vi "SubPanel - Power Analysis.vi"() -> ()   [LabVIEW 2021]
uses:
  <vilib>/Analysis/5stat.llb/RMS (DBL).vi
  <vilib>/Analysis/NI_AALPro.lvlib
panel:
  out "error out":errorcluster
  in  "error in":errorcluster
  in  "Samples per Channel":i32
  out "I Phase L3":dbl format="%#.3g"
  out "I Phase L2":dbl format="%#.3g"
  out "I Phase L1":dbl format="%#.3g"
  out "Instantaneus Currents":dbl[][](graph)
  out "P/S Total":dbl format="%#.3g"
  out "Q Total":dbl format="%#.3f"
  out "P Total":dbl format="%#.3g"
  out "S Total":dbl format="%#.3g"
  out "Power Values Phase L3":T1 {"Power Factor P/S" format="%#.3g"; "Reactive Power Q" format="%#.3g"; "Active Power P" format="%#.3g"; "Apparent Power S" format="%#.3g"}
  out "Power Values Phase L2":T1 {"Power Factor P/S" format="%#.3g"; "Reactive Power Q" format="%#.3g"; "Active Power P" format="%#.3g"; "Apparent Power S" format="%#.3g"}
  out "Power Values Phase L1":T1 {"Power Factor P/S" format="%#.3g"; "Reactive Power Q" format="%#.3f"; "Active Power P" format="%#.3g"; "Apparent Power S" format="%#.3g"}
  out "U Phase L3":dbl format="%#.3g"
  out "U Phase L2":dbl format="%#.3g"
  out "U Phase L1":dbl format="%#.3g"
  out "Instantaneus Voltages":dbl[][](graph)
  # "V"
  # "V"
  # "V"
  # "A"
  # "A"
  # "A"
  # "RMS Values"
  # "RMS Values"
  # "Powers Values Phase L1"
  # "kVA"
  # "kW"
  # "Powers Values Phase L2"
  # "kVAr"
  # "Powers Values Phase L3"
  # "VA"
  # "W"
  # "VAr"
  # "VA"
  # "W"
  # "VAr"
  # "VA"
  # "W"
  # "VAr"
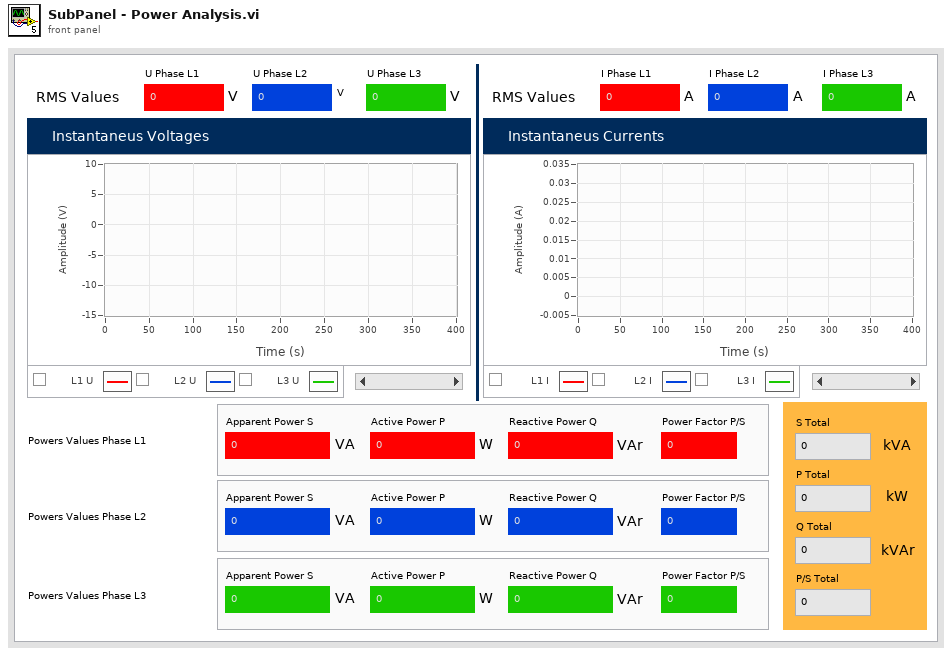
[diagram p1: front panel]
types:
  T1 = cluster{"Apparent Power S":dbl, "Active Power P":dbl, "Reactive Power Q":dbl, "Power Factor P/S":dbl}
  T2 = typedef "Message FPGA.ctl" = cluster{"Channel 1 Data (L1 U)":dbl[], "Channel 2 Data (L1 I)":dbl[], "Channel 3 Data (L2 U)":dbl[], "Channel 4 Data (L2 I)":dbl[], "Channel 5 Data (L3 U)":dbl[], "Channel 6 Data (L3 I)":dbl[]}
  T3 = typedef "Powers Values.ctl" = cluster{"Apparent Power S [VA]":dbl, "Active Power P [W]":dbl, "Reactive Power Q [var]":dbl, "Power Factor P/S":dbl}
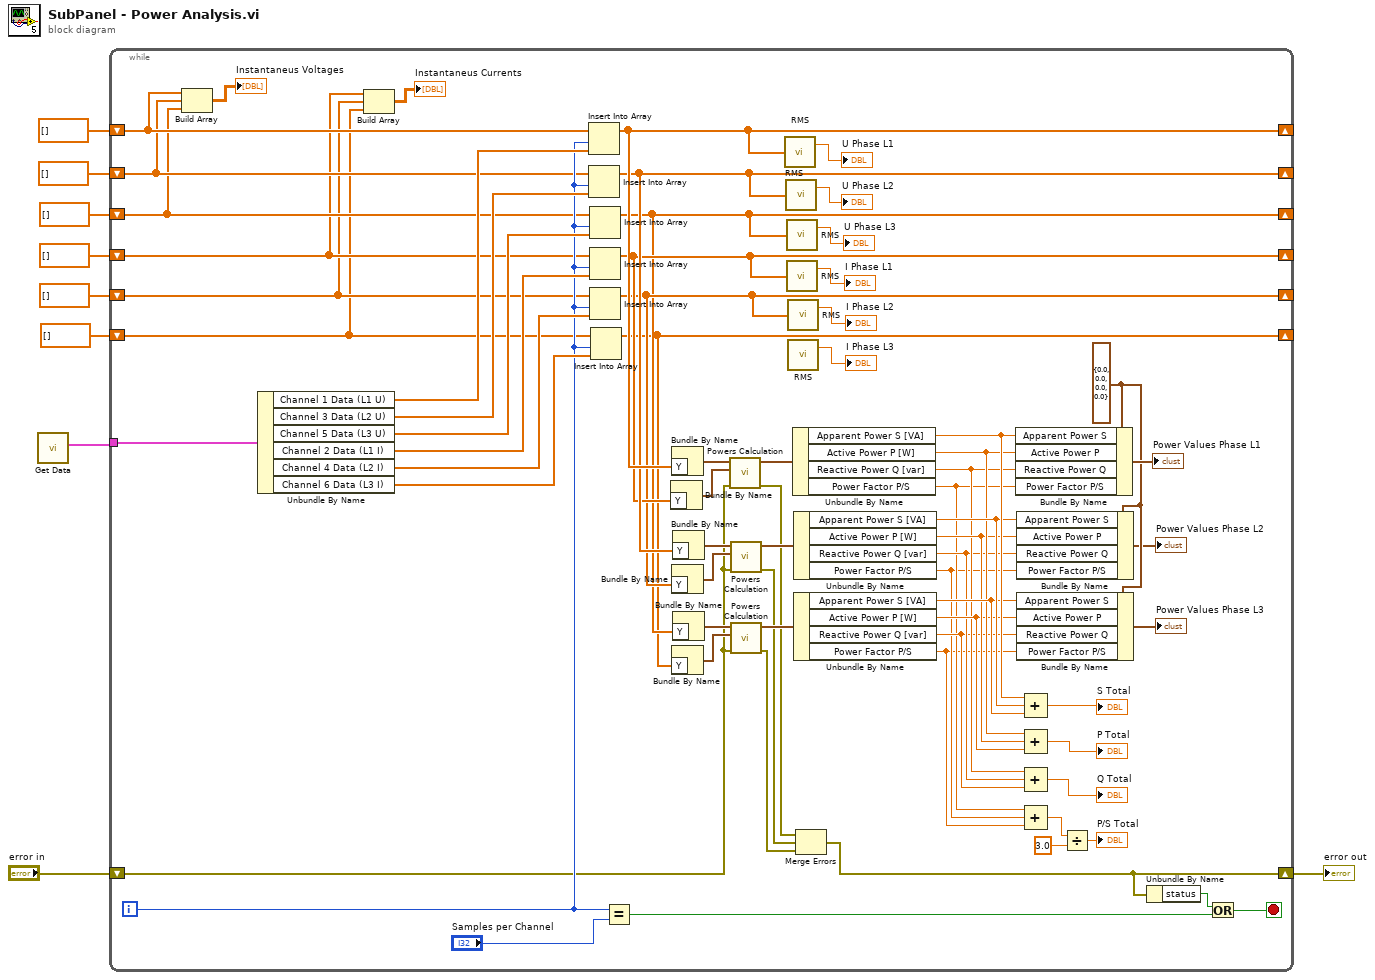
[diagram p0: block diagram]
diagram:
  n1 = call "Get Data.vi"() -> ("Message FPGA"=w1:T2)  [unwired: 10 in, 1 out]
  n2 = while {
    tunnel: w1 -> [w77]
    shift-right: [w48] -> _
    shift-left: dbl[] [] -> [w63]
    shift-right: [w37] -> _
    shift-left: dbl[] [] -> [w62]
    shift-right: [w34] -> _
    shift-left: dbl[] [] -> [w61]
    shift-right: [w36] -> _
    shift-left: dbl[] [] -> [w60]
    shift-right: [w35] -> _
    shift-left: dbl[] [] -> [w59]
    shift-right: [w33] -> _
    shift-left: dbl[] [] -> [w58]
    shift-right: [w10] -> w2
    shift-left: "error in" -> [w14]
    i -> [w70]
    stop <- w68 stop-if-true
    w40 = T1 {"Apparent Power S"=0.0, "Active Power P"=0.0, "Reactive Power Q"=0.0, "Power Factor P/S"=0.0} ("Power Values Phase L1")
    n3 = Build Array(w63, w62, w61) -> (→"Instantaneus Voltages":dbl[][])
    n4 = Unbundle By Name(w77) -> ("Channel 1 Data (L1 U)"=w76:dbl[], "Channel 3 Data (L2 U)"=w75:dbl[], "Channel 5 Data (L3 U)"=w74:dbl[], "Channel 2 Data (L1 I)"=w73:dbl[], "Channel 4 Data (L2 I)"=w72:dbl[], "Channel 6 Data (L3 I)"=w71:dbl[])
    n5 = Build Array(w60, w59, w58) -> (→"Instantaneus Currents":dbl[][])
    n6 = Insert Into Array(array=w63, index=w70, new element=w76) -> (w48:dbl[])
    n7 = Insert Into Array(array=w62, index=w70, new element=w75) -> (w37:dbl[])
    n8 = Insert Into Array(array=w61, index=w70, new element=w74) -> (w34:dbl[])
    n9 = Insert Into Array(array=w60, index=w70, new element=w73) -> (w36:dbl[])
    n10 = Insert Into Array(array=w59, index=w70, new element=w72) -> (w35:dbl[])
    n11 = Insert Into Array(array=w58, index=w70, new element=w71) -> (w33:dbl[])
    n12 = Equal?(x=w70, y="Samples per Channel") -> (x = y?=w66:bool)
    n13 = Bundle By Name("Y"=w36) -> (w44:waveform(dbl))  [unwired: 1 in]
    n14 = Bundle By Name("Y"=w48) -> (w51:waveform(dbl))  [unwired: 1 in]
    n15 = Bundle By Name("Y"=w35) -> (w46:waveform(dbl))  [unwired: 1 in]
    n16 = Bundle By Name("Y"=w33) -> (w42:waveform(dbl))  [unwired: 1 in]
    n17 = Bundle By Name("Y"=w37) -> (w45:waveform(dbl))  [unwired: 1 in]
    n18 = Bundle By Name("Y"=w34) -> (w43:waveform(dbl))  [unwired: 1 in]
    n19 = call "Powers Calculation.vi"("Error In"=w14, "Voltage Waveform"=w44, "Current Waveform"=w51) -> ("Error Out"=w13:errorcluster, "Power Values"=w50:T3)  [unwired: 7 in]
    n20 = call "Powers Calculation.vi"("Error In"=w14, "Voltage Waveform"=w46, "Current Waveform"=w45) -> ("Error Out"=w12:errorcluster, "Power Values"=w47:T3)  [unwired: 7 in]
    n21 = call "Powers Calculation.vi"("Error In"=w14, "Voltage Waveform"=w42, "Current Waveform"=w43) -> ("Error Out"=w11:errorcluster, "Power Values"=w41:T3)  [unwired: 7 in]
    n22 = call-poly <vilib>:"RMS.vi"("X"=w48) -> ("rms value"=→"U Phase L1":dbl)  [unwired: 1 out]
    n23 = call-poly <vilib>:"RMS.vi"("X"=w37) -> ("rms value"=→"U Phase L2":dbl)  [unwired: 1 out]
    n24 = call-poly <vilib>:"RMS.vi"("X"=w34) -> ("rms value"=→"U Phase L3":dbl)  [unwired: 1 out]
    n25 = call-poly <vilib>:"RMS.vi"("X"=w36) -> ("rms value"=→"I Phase L1":dbl)  [unwired: 1 out]
    n26 = call-poly <vilib>:"RMS.vi"("X"=w35) -> ("rms value"=→"I Phase L2":dbl)  [unwired: 1 out]
    n27 = call-poly <vilib>:"RMS.vi"() -> ("rms value"=→"I Phase L3":dbl)  [unwired: 1 in, 1 out]
    n28 = Unbundle By Name(w50) -> ("Apparent Power S [VA]"=w29:dbl, "Active Power P [W]"=w25:dbl, "Reactive Power Q [var]"=w21:dbl, "Power Factor P/S"=w18:dbl)
    n29 = Unbundle By Name(w47) -> ("Apparent Power S [VA]"=w28:dbl, "Active Power P [W]"=w24:dbl, "Reactive Power Q [var]"=w20:dbl, "Power Factor P/S"=w17:dbl)
    n30 = Unbundle By Name(w41) -> ("Apparent Power S [VA]"=w27:dbl, "Active Power P [W]"=w23:dbl, "Reactive Power Q [var]"=w19:dbl, "Power Factor P/S"=w16:dbl)
    n31 = Merge Errors(w13, w12, w11) -> (w10:errorcluster)
    n32 = Bundle By Name(cluster=w40, "Apparent Power S"=w29, "Active Power P"=w25, "Reactive Power Q"=w21, "Power Factor P/S"=w18) -> (→"Power Values Phase L1":T1)
    n33 = Bundle By Name(cluster=w40, "Apparent Power S"=w28, "Active Power P"=w24, "Reactive Power Q"=w20, "Power Factor P/S"=w17) -> (→"Power Values Phase L2":T1)
    n34 = Bundle By Name(cluster=w40, "Apparent Power S"=w27, "Active Power P"=w23, "Reactive Power Q"=w19, "Power Factor P/S"=w16) -> (→"Power Values Phase L3":T1)
    n35 = Compound Arithmetic op=ADD(w29, w28, w27) -> (→"S Total":dbl)
    n36 = Compound Arithmetic op=ADD(w25, w24, w23) -> (→"P Total":dbl)
    n37 = Compound Arithmetic op=ADD(w21, w20, w19) -> (→"Q Total":dbl)
    n38 = Compound Arithmetic op=ADD(w18, w17, w16) -> (w31:dbl)
    n39 = Divide(x=w31, y=3.0) -> (x/y=→"P/S Total":dbl)
    n40 = Unbundle By Name(w10) -> ("status"=w67:bool)
    n41 = Or(x=w67, y=w66) -> (x .or. y?=w68:bool)
  }
  "error out" <- w2
